vi "StahlPS_Pbus.ProcEvents.vi"(0 "i ref in":refnum<vi>, 5 "error in":errorcluster) -> (14 "i ref out":refnum<vi>, 19 "error out":errorcluster)   [LabVIEW 2014, in "StahlPS_Pbus.lvlib"]
doc: "This method is used to define the events the object will listen to. Add your own events here."
uses:
  StahlPS_Pbus.lvlib
  CSCore/BaseProcess/BaseProcess.event definition.ctl
  CSCore/CAEObj/CAEObj.event definition.ctl
  CSCore/BaseProcess/BaseProcess.descriptor string definition.ctl
  CSCore/BaseProcess/BaseProcess.lvlib
  CSCore/CAEObj/CAEObj.lvlib
  CSCore/CSSystem/CSSystemLib/CSSystemLib.lvlib
panel:
  in  "dummy":T1
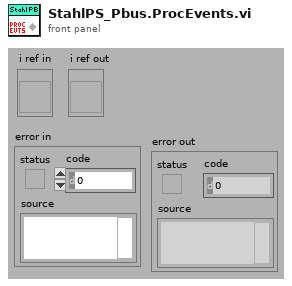
[diagram p1: front panel]
types:
  T1 = typedef "BaseProcess.lvlib/BaseProcess.event definition.ctl" = cluster{"CAEEvtDef":T2, "Data Descriptor":T3}
  T2 = typedef "CAEObj.lvlib/CAEObj.event definition.ctl" = cluster{"URL":string, "enable":bool, "ignoreResID":bool}
  T3 = typedef "BaseProcess.lvlib/BaseProcess.descriptor string definition.ctl" = string
  T4 = typedef "StahlPS_Pbus.lvlib/StahlPS_Pbus.i attribute.ctl" = cluster{"Type":string, "CALC_FACTOR_SET_VOLTAGE":dbl, "CALC_FACTOR_GET_VOLTAGE":dbl, "CALC_FACTOR_GET_CURRENT":dbl, "CALC_FACTOR_SET_CURRENT ":dbl, "REG_VALUE":dbl, "Sign":bool, "setVoltIDs":i32[], "Elektrode Names":string[]}
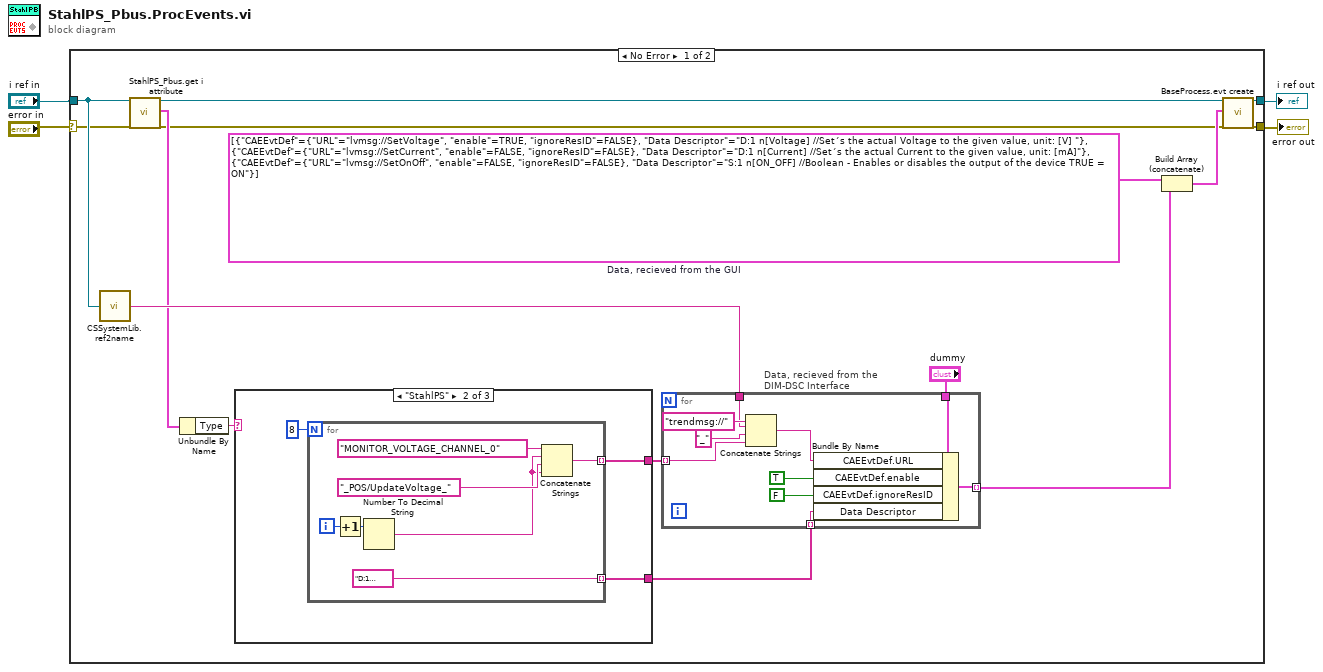
[diagram p0: block diagram]
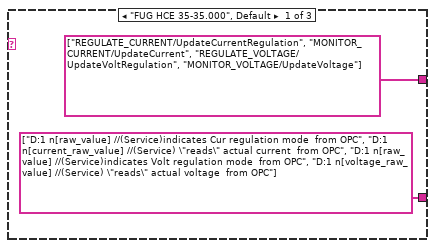
[diagram p2: hidden frame]
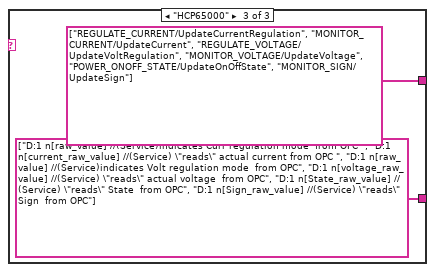
[diagram p3: hidden frame]
diagram:
  n1 = case shown="No Error" "error in" {
    selector: "error in" -> [w8 w44]
    tunnel: "i ref in" -> [w10 w45]
    tunnel: [w15 w45] -> w2
    tunnel: [w19 w44] -> w1
    frame No Error {
      w16 = T1[] [{"CAEEvtDef"={"URL"="lvmsg://SetVoltage", "enable"=TRUE, "ignoreResID"=FALSE}, "Data Descriptor"="D:1 n[Voltage] //Set´s the actual Voltage to the given value, unit: [V] "}, {"CAEEvtDef"={"URL"="lvmsg://SetCurrent", "enable"=FALSE, "ignoreResID"=FALSE}, "Data Descriptor"="D:1 n[Current] //Set´s the actual Current to the given value, unit: [mA]"}, {"CAEEvtDef"={"URL"="lvmsg://SetOnOff", "enable"=FALSE, "ignoreResID"=FALSE}, "Data Descriptor"="S:1 n[ON_OFF] //Boolean - Enables or disables the output of the device TRUE = ON"}]  # Data, recieved from the GUI
      n2 = call "CSSystemLib.ref2name.vi"("obj refnum"=w10) -> ("name"=w12:string)
      n3 = call "StahlPS_Pbus.get i attribute.vi"("i ref in"=w10, "error in (no error)"=w8) -> ("i ref out"=w9:refnum<vi>, "i attribute"=w11:T4, "error out"=w7:errorcluster)  [unwired: 15 in]
      n4 = Unbundle By Name(w11) -> ("Type"=w6:string)
      n5 = case shown="\"StahlPS\"" w6 {
        tunnel: [string[] ["REGULATE_CURRENT/UpdateCurrentRegulation", "MONITOR_CURRENT/UpdateCurrent", "REGULATE_VOLTAGE/UpdateVoltRegulation", "MONITOR_VOLTAGE/UpdateVoltage"] w22 string[] ["REGULATE_CURRENT/UpdateCurrentRegulation", "MONITOR_CURRENT/UpdateCurrent", "REGULATE_VOLTAGE/UpdateVoltRegulation", "MONITOR_VOLTAGE/UpdateVoltage", "POWER_ONOFF_STATE/UpdateOnOffState", "MONITOR_SIGN/UpdateSign"]] -> w14
        tunnel: [string[] ["D:1 n[raw_value] //(Service)indicates Cur regulation mode  from OPC", "D:1 n[current_raw_value] //(Service) \"reads\" actual current  from OPC", "D:1 n[raw_value] //(Service)indicates Volt regulation mode  from OPC", "D:1 n[voltage_raw_value] //(Service) \"reads\" actual voltage  from OPC"] w24 string[] ["D:1 n[raw_value] //(Service)indicates Curr regulation mode  from OPC ", "D:1 n[current_raw_value] //(Service) \"reads\" actual current from OPC ", "D:1 n[raw_value] //(Service)indicates Volt regulation mode  from OPC", "D:1 n[voltage_raw_value] //(Service) \"reads\" actual voltage  from OPC", "D:1 n[State_raw_value] //(Service) \"reads\" State  from OPC", "D:1 n[Sign_raw_value] //(Service) \"reads\" Sign  from OPC"]] -> w5
        frame "FUG HCE 35-35.000", Default {
        }
        frame "StahlPS" {
          n6 = for {
            N: 8 -> [_]
            tunnel: ["D:1 n[voltage_raw_value] //(Service) \"reads\" actual voltage from OPC"] -> w24 mode=indexing
            tunnel: [w25] -> w22 mode=indexing
            i -> [w28]
            n7 = Increment(x=w28) -> (x+1=w27:i32)
            n8 = Number To Decimal String(number=w27) -> (decimal integer string=w26:string)  [unwired: 1 in]
            n9 = Concatenate Strings("MONITOR_VOLTAGE_CHANNEL_0", w26, "_POS/UpdateVoltage_", w26) -> (w25:string)
          }
        }
        frame "HCP65000" {
        }
      }
      n10 = for "Data, recieved from the DIM-DSC Interface" {
        tunnel: "dummy" -> [w43]
        tunnel: [w40] -> w13 mode=indexing
        tunnel: w12 -> [w37]
        tunnel: w14 -> [w36] mode=indexing
        tunnel: w5 -> [w34] mode=indexing
        n11 = Concatenate Strings("trendmsg://" ("string"), w37, "_" ("string"), w36) -> (w35:string)
        n12 = Bundle By Name(cluster=w43, "CAEEvtDef.URL"=w35, "CAEEvtDef.enable"=TRUE, "CAEEvtDef.ignoreResID"=FALSE, "Data Descriptor"=w34) -> (w40:T1)
      }
      n13 = Build Array (concatenate)(w16, w13) -> (w17:T1[])
      n14 = call "BaseProcess.evt create.vi"("i ref in"=w9, "newEvents"=w17, "error in (no error)"=w7) -> ("i ref out"=w15:refnum<vi>, "error out"=w19:errorcluster)  [unwired: 13 in, 2 out]
    }
    frame Error {
    }
  }
  "i ref out" <- w2
  "error out" <- w1
